vi "Engine.vi"(5 "error in":errorcluster, 6 "Other Outputs":cluster{"Alarm":bool, "Heater":bool}, 7 "Final Output Controls":T2, 8 "Com Parms":T1={"VISA resource name"="COM3", "baud rate"=38400, "data bits"=8, "parity"=0, "stop bits"=10, "flow control"=0} {"flow control" items=["None"=0, "XON/XOFF"=1, "RTS/CTS"=2, "DTR/DSR"=4]; "stop bits" items=["1.0"=10, "1.5"=15, "2.0"=20]; "parity" items=["None", "Odd", "Even", "Mark", "Space"]; "data bits" min=5 max=8 step=1}) -> (0 "error out":errorcluster, 3 "Data Read":T3={"Date"="03/13/13", "Time"="48:48:32", "CO2- ppm"=533, "Last Ctrl Word"=400000, "O2-1 ppm"=208865, "O2-2 ppm"=208845, "Temp MB"=18.59, "Temp Sensor Module"=21.2, "Press mB"=840.1} {"Last Ctrl Word" format="%.0x"})   [LabVIEW 2012]
uses:
  Type Defs/Final Output for Dispaly.ctl
panel:
  # "W/R from\nControl Change"
  # "Channel A"
  # "Channel B"
  # "Channel C"
  # "Channel D"
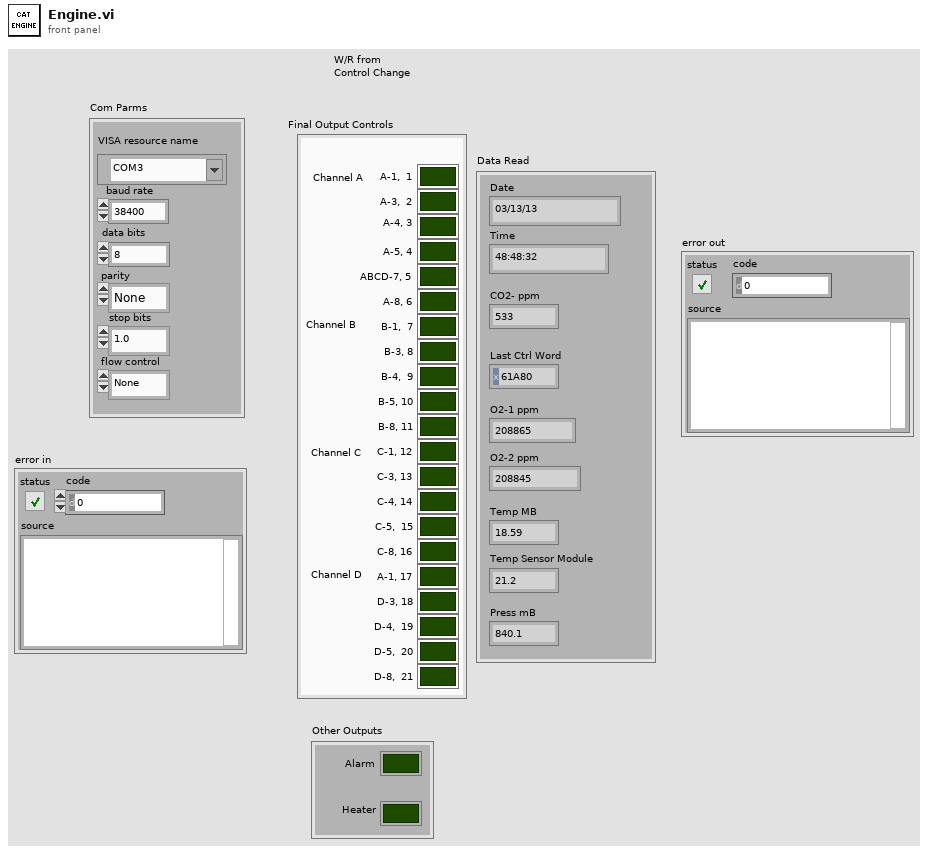
[diagram p1: front panel]
types:
  T1 = cluster{"VISA resource name":refnum<visa-resource-name>, "baud rate":u32, "data bits":u16, "parity":u16, "stop bits":u16, "flow control":u16}
  T2 = typedef "Final Output for Dispaly.ctl" = cluster{"A-1,  1":bool, "A-3,  2":bool, "A-4, 3":bool, "A-5, 4":bool, "ABCD-7, 5":bool, "A-8, 6":bool, "B-1,  7":bool, "B-3, 8":bool, "B-4,  9":bool, "B-5, 10":bool, "B-8, 11":bool, "C-1, 12":bool, "C-3, 13":bool, "C-4, 14":bool, "C-5,  15":bool, "C-8, 16":bool, "A-1, 17":bool, "D-3, 18":bool, "D-4,  19":bool, "D-5,  20":bool, "D-8,  21":bool}
  T3 = cluster{"Date":string, "Time":string, "CO2- ppm":u32, "Last Ctrl Word":u32, "O2-1 ppm":u32, "O2-2 ppm":u32, "Temp MB":sgl, "Temp Sensor Module":sgl, "Press mB":sgl}
  T4 = cluster{"Date":string, "Time":string, "CO2- ppm":u32, "Last Ctrl Word":u32, "O2-1 ppm":u32, "O2-2 ppm":u32, "Temp MB":sgl, "Temp Sensor Modulr":sgl, "Press mB":sgl}
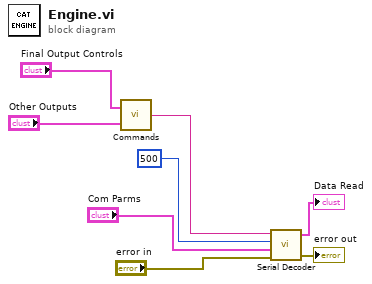
[diagram p0: block diagram]
diagram:
  n1 = call "Commands.vi"("Final Output"="Final Output Controls", "Other Outputs"="Other Outputs") -> ("hex integer string"=w1:string)  [unwired: 2 out]
  n2 = call "Serial Decoder.vi"("Write Value"=w1, "milliseconds to wait"=u32 500, "Com Parms"="Com Parms", "error in"="error in") -> ("Data Read"=→"Data Read":T4, "error out"=→"error out":errorcluster)  [unwired: 2 in]
